vi "SubscribedMessages.vi"() -> (3 "subscribed messages":string[](array[string]))   [LabVIEW 2017, in "Trigger.lvlib"]
uses:
  <vilib>/addons/InsightCM/Devices/Shared/Common/Trigger/Trigger.lvlib
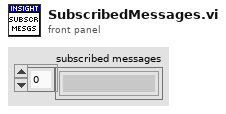
[diagram p1: front panel]
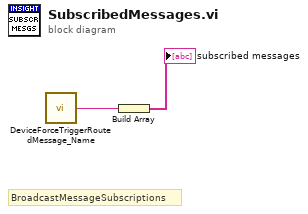
[diagram p0: block diagram]
diagram:
  # "BroadcastMessageSubscriptions"
  n1 = call <vilib>:"DeviceForceTriggerRoutedMessage_Name.vi"() -> ("MessageName"=w2:string)  [unwired: 5 in]
  n2 = Build Array(w2) -> (→"subscribed messages":string[])
